vi "delete alarm.vi"(8 "error in":errorcluster, 10 "alarm name":string, 11 "alarms module configuration in":refnum<class "alarms module configuration.lvclass">) -> (0 "error out":errorcluster, 2 "deleted channels":refnum<class "TBM channel.lvclass">[](array[class]), 3 "alarms module configuration out":refnum<class "alarms module configuration.lvclass">)   [LabVIEW 2013, in "alarms module configuration.lvclass"]
uses:
  alarms module configuration.lvclass
  <vilib>/NI/Tag Bus Module Framework/channel/TBM channel.lvclass
  alarms module configuration.lvclass/alarms module configuration.ctl
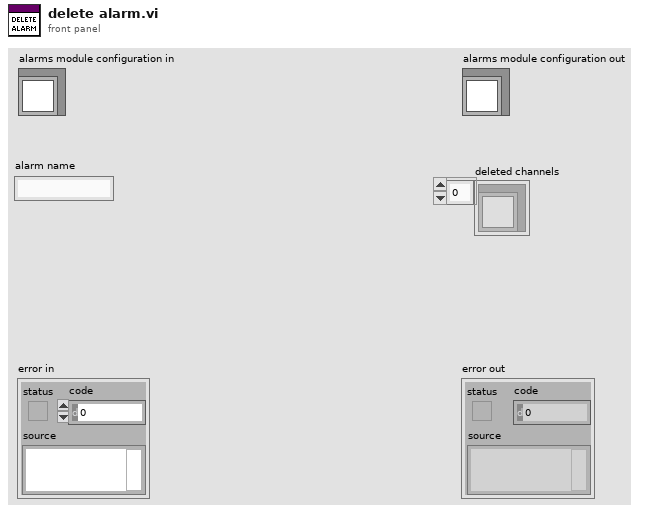
[diagram p1: front panel]
types:
  T1 = typedef "alarms module configuration.lvclass/alarm configuration.ctl" = cluster{"alarm name":string, "comparisons":T2[], "unlatch":refnum<class "TBM channel.lvclass">, "output":refnum<class "TBM channel.lvclass">, "boolean op":T4}
  T2 = typedef "alarms module configuration.lvclass/alarm comparison.ctl" = cluster{"input channel":refnum<class "TBM channel.lvclass">, "limit":dbl, "comparison":T3}
  T3 = typedef "alarms module configuration.lvclass/compare type.ctl" = enum16{">", "<", ">=", "<=", "="}
  T4 = typedef "alarms module configuration.lvclass/boolean operation.ctl" = enum16{"AND", "OR"}
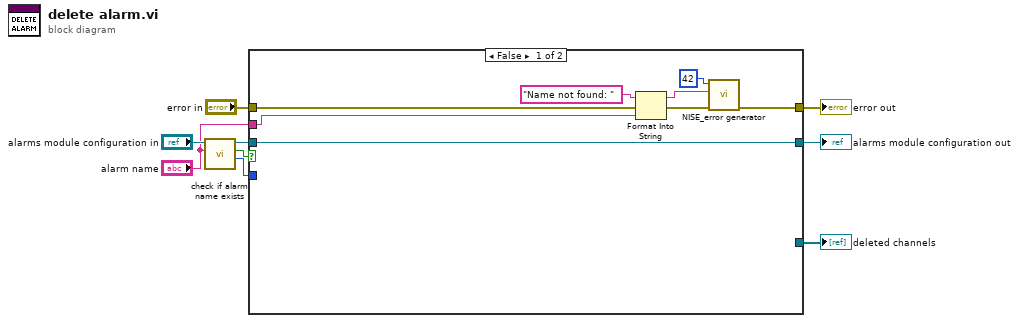
[diagram p0: block diagram]
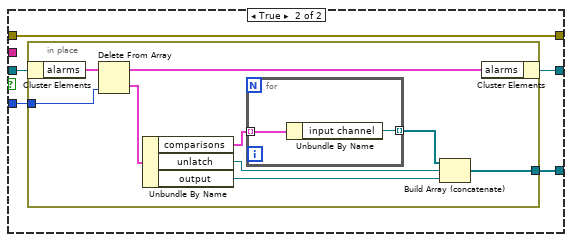
[diagram p2: hidden frame]
diagram:
  n1 = call "check if alarm name exists.vi"("name to locate"="alarm name", "alarms module configuration in"="alarms module configuration in") -> ("index"=w2:i32, "found?"=w6:bool, "alarms module configuration out"=w4:refnum<class "alarms module configuration.lvclass">)  [unwired: 7 in]
  n2 = case shown="False" w6 {
    tunnel: [w16 w20] -> w8
    tunnel: "error in" -> [w17 w20]
    tunnel: [w11 w21] -> w5
    tunnel: w4 -> [w11 w22]
    tunnel: [_ w19] -> w3
    tunnel: w2 -> [_ w18]
    tunnel: "alarm name" -> [w10 _]
    frame False {
      n3 = Format Into String(initial string="Name not found: " ("append error message"), error in=w17, w10) -> (resulting string=w12:string, error out=w14:errorcluster)  [unwired: 1 in]
      n4 = call <vilib>:"NISE_error generator.vi"("error in"=w14, "append error message"=w12, "error code (0)"=42) -> ("error out"=w16:errorcluster)  [unwired: 6 in]
    }
    frame True {
      n5 = in-place {
        in-place-border: [w25] -> w19
        in-place-border: w18 -> [w29]
        n6 = in-place-cluster #1(w22) -> ("alarms"=w31:T1[])
        n7 = Delete From Array(array=w31, index=w29) -> (deleted portion=w28:T1, array with subset deleted=w30:T1[])  [unwired: 1 in]
        n8 = Unbundle By Name(w28) -> ("comparisons"=w27:T2[], "unlatch"=w24:refnum<class "TBM channel.lvclass">, "output"=w23:refnum<class "TBM channel.lvclass">)
        n9 = for {
          tunnel: w27 -> [w33] mode=indexing
          tunnel: [w32] -> w26 mode=indexing
          n10 = Unbundle By Name(w33) -> ("input channel"=w32:refnum<class "TBM channel.lvclass">)
        }
        n11 = Build Array (concatenate)(w26, w24, w23) -> (w25:refnum<class "TBM channel.lvclass">[])
        n12 = in-place-cluster #1("alarms"=w30) -> (w21:refnum<class "alarms module configuration.lvclass">)
      }
    }
  }
  "error out" <- w8
  "alarms module configuration out" <- w5
  "deleted channels" <- w3
